vi "CreateBodyText.vi"(9 "Body Text":T2={"Line 1 text"="", "Line 2 text"="", "Line 3 text"="", "Line 4 text"="", "Line 1 color"=0, "Line 2 color"=0, "Line 3 color"=0, "Line 4 color"=0, "Body Text Spec"={"Font"="", "Alignment"=0, "Size"=3}, "Center text vertically"=FALSE, "Capitalize Text"=FALSE} {"Body Text Spec"."Alignment" items=["left", "center", "right"]}, 10 "Path and Icon Template":T1, 11 "Icon.lvclass in":refnum<class "Icon.lvclass">) -> (1 "Body Text":picture)   [LabVIEW 2017, in "Icon Framework.lvclass"]
doc: "The incoming style information and actual text is used to actually create a picture."
uses:
  <vilib>/LabVIEW Icon API/lv_icon/Classes/Icon Framework/Icon Framework.lvclass
  <vilib>/LabVIEW Icon API/lv_icon/Controls/BodyText.ctl
  <vilib>/LabVIEW Icon API/lv_icon/Controls/Font.ctl
  <vilib>/LabVIEW Icon API/lv_icon/Controls/Alignment.ctl
  <vilib>/LabVIEW Icon API/lv_icon/Classes/Icon/Icon.lvclass
  <vilib>/LabVIEW Icon API/lv_icon/Controls/Graphic.ctl
  <vilib>/LabVIEW Icon API/lv_icon/lv_icon.lvlib
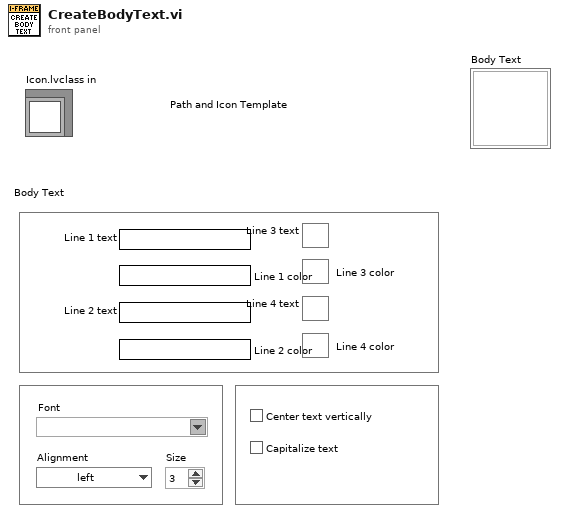
[diagram p1: front panel]
types:
  T1 = typedef "Graphic.ctl" = cluster{"Rectangle":cluster{"left":i16, "top":i16, "right":i16, "bottom":i16}, "Path":path, "Image":picture, "Filter":string, "FileName":string}
  T2 = typedef "BodyText.ctl" = cluster{"Line 1 text":string, "Line 2 text":string, "Line 3 text":string, "Line 4 text":string, "Line 1 color":u32, "Line 2 color":u32, "Line 3 color":u32, "Line 4 color":u32, "Body Text Spec":cluster{"Font":T3, "Alignment":T4, "Size":u8}, "Center text vertically":bool, "Capitalize Text":bool}
  T3 = typedef "Font.ctl" = string
  T4 = typedef "Alignment.ctl" = u16
  T5 = cluster{"Font Name:":string, "Size":i16, "Strikeout?":bool, "Italic?":bool, "Underline?":bool, "Outline?":bool, "Shadow?":bool, "Bold?":bool}
  T6 = cluster{"horizontal":enum16{"left", "center", "right"}, "vertical":enum16{"top", "center", "bottom"}}
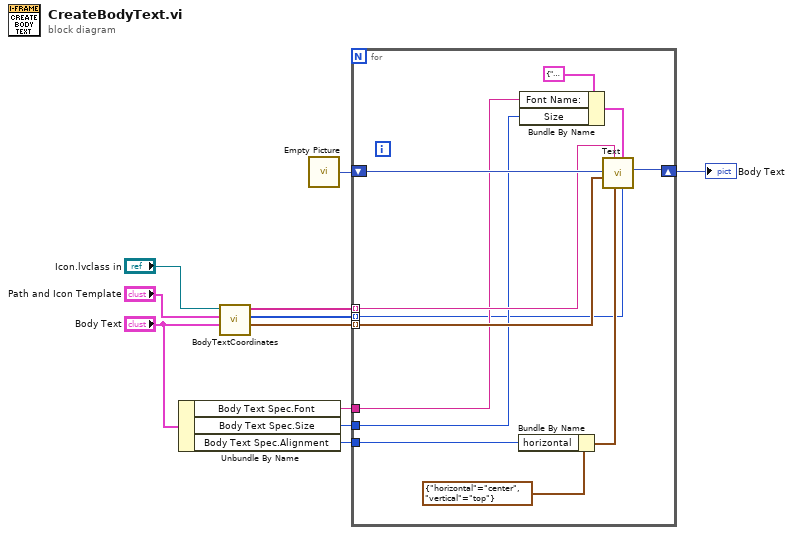
[diagram p0: block diagram]
diagram:
  n1 = Unbundle By Name("Body Text") -> ("Body Text Spec.Font"=w5:T3, "Body Text Spec.Size"=w4:u8, "Body Text Spec.Alignment"=w6:T4)
  n2 = call <vilib>:"BodyTextCoordinates.vi"("Body Text"="Body Text", "Path and Icon Template"="Path and Icon Template", "Icon.lvclass in"="Icon.lvclass in") -> ("Coordinates"=w9:cluster{"x":i16, "y":i16}[], "color out"=w7:u32[], "Lines out"=w8:string[])  [unwired: 5 in, 1 out]
  n3 = call "Empty Picture"() -> ("empty picture"=w11:picture)
  n4 = for {
    tunnel: w6 -> [w23]
    shift-right: [w18] -> w10
    shift-left: w11 -> [w17]
    tunnel: w8 -> [w15] mode=indexing
    tunnel: w9 -> [w16] mode=indexing
    tunnel: w4 -> [w13]
    tunnel: w5 -> [w14]
    tunnel: w7 -> [w12] mode=indexing
    n5 = Bundle By Name(cluster=T6 {"horizontal"=enum."center", "vertical"=enum."top"} ("alignment(left, top)"), "horizontal"=w23) -> (w20:T6)
    n6 = Bundle By Name(cluster=T5 {"Font Name:"="", "Size"=12, "Strikeout?"=FALSE, "Italic?"=FALSE, "Underline?"=FALSE, "Outline?"=FALSE, "Shadow?"=FALSE, "Bold?"=FALSE} ("[user-specified font]"), "Font Name:"=w14, "Size"=w13) -> (w19:T5)
    n7 = call <vilib>:"Text.vi"("text color(black)"=w12, "[user-specified font]"=w19, "alignment(left, top)"=w20, "text"=w15, "origin"=w16, "picture"=w17) -> ("new picture"=w18:picture)  [unwired: 4 in, 1 out]
  }
  "Body Text" <- w10
